vi "CreateErrorValue.vi"(9 "Status (true=error)":bool=TRUE, 10 "Source Prefix":string, 11 "Error Number":i32) -> (3 "output cluster":errorcluster)   [LabVIEW 2013, in "BarCodes.lvlib"]
uses:
  BarCodes.lvlib
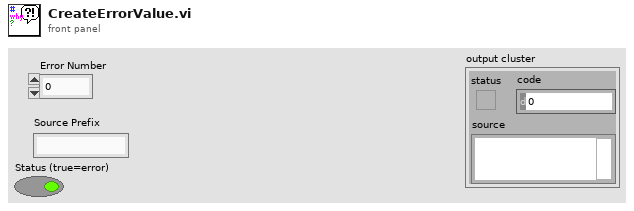
[diagram p1: front panel]
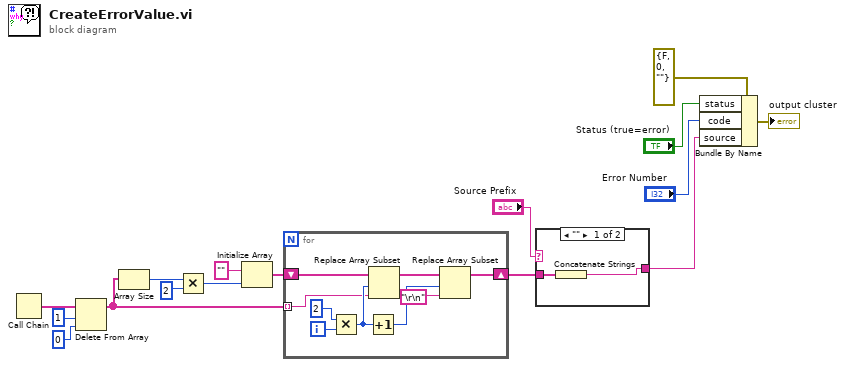
[diagram p0: block diagram]
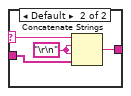
[diagram p2: hidden frame]
diagram:
  n1 = Call Chain() -> (call chain=w16:string[])
  n2 = Delete From Array(array=w16, length=1, index=0) -> (array with subset deleted=w7:string[])  [unwired: 1 out]
  n3 = Array Size(array=w7) -> (size(s)=w12:i32)
  n4 = Multiply(x=w12, y=2) -> (x*y=w10:i32)
  n5 = Initialize Array("" ("Source Prefix"), w10) -> (w9:string[])
  n6 = for {
    shift-right: [w18] -> w8
    shift-left: w9 -> [w25]
    tunnel: w7 -> [w17] mode=indexing
    i -> [w23]
    n7 = Multiply(x=2, y=w23) -> (x*y=w21:i32)
    n8 = Increment(x=w21) -> (x+1=w20:i32)
    n9 = Replace Array Subset(array=w25, new element=w17, index=w21) -> (w22:string[])
    n10 = Replace Array Subset(array=w22, new element="\r\n", index=w20) -> (w18:string[])
  }
  n11 = case shown="\"\"" "Source Prefix" {
    selector: "Source Prefix" -> [_ w28]
    tunnel: w8 -> [w27 w30]
    tunnel: [w26 w29] -> w3
    frame "" {
      n12 = Concatenate Strings(w27) -> (w26:string)
    }
    frame Default {
      w31 = "\r\n"
      n13 = Concatenate Strings(w28, w31, w31, w30) -> (w29:string)
    }
  }
  n14 = Bundle By Name(cluster=errorcluster {"status"=FALSE, "code"=0, "source"=""} ("error constant"), "status"="Status (true=error)", "code"="Error Number", "source"=w3) -> (→"output cluster":errorcluster)
